vi "Test of XiXi-1.vi"() -> ()   [LabVIEW 2011]
panel:
  in  "X[-1]":dbl
  in  "Xi":dbl[](array[numeric])
  out "Yi":dbl[][](array[numeric])
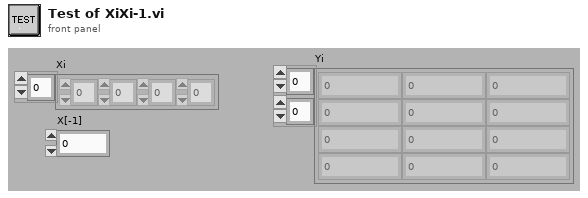
[diagram p1: front panel]
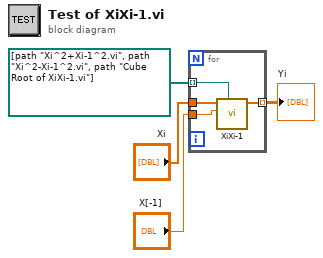
[diagram p0: block diagram]
diagram:
  n1 = for {
    tunnel: "X[-1]" -> [w8]
    tunnel: path[] [path "Xi^2+Xi-1^2.vi", path "Xi^2-Xi-1^2.vi", path "Cube Root of XiXi-1.vi"] -> [w7] mode=indexing
    tunnel: "Xi" -> [w6]
    tunnel: [w5] -> w1 mode=indexing
    n2 = call "XiXi-1.vi"("VI路径"=w7, "X[-1]"=w8, "Xi"=w6) -> ("Yi"=w5:dbl[])  [unwired: 8 in]
  }
  "Yi" <- w1
